vi "DP Analysis Panel.vi"(9 "Autosave? (F)":bool, 11 "Data folder in":path) -> ()   [LabVIEW 2020]
uses:
  epl-vi-lib/Utility VIs/Controls/KLegend/KLegend.xctl
  Typedefs/DP-Comparison List.ctl
  <vilib>/regexp/Match Regular Expression.xnode
panel:
  out "IOLeg":dbl(xcontrol)
  in  "Tab Control":enum32{"Isoresponse", "DP vs F2"}(tab)
  out "DPGram":cluster{"I-O Plot":dbl[], "I-O Plot":dbl[]}[](graph)
  out "DPvsFreq":cluster{"I-O Plot":dbl[], "I-O Plot":dbl[]}[](graph)
  out "DPvsF2Leg":dbl(xcontrol)
  out "exit signal":bool
  in  "Save programatically":bool
  in  "Analysis mode":enum32{"Browse", "Compare"}(tab)=enum."Compare"
  in  "Compare>":bool
  in  "File list":i32[](listbox)
  in  "Save":bool
  in  "Data folder":path
  in  "Compare list":i32[](listbox)=[0]
  in  "Criterion (dB SPL)":u16(ring)=1 items=["-5", "0", "5", "10", "15", "20", "25"]
  in  "F2 (kHz)":u16(ring) items=["5645.70", "7995.60", "11322.00", "15991.00", "22644.00", "32012.00", "45257.00", "3997.80", "5615.20", "11291.00", "22613.00"]
  in  "Exit":bool
  out "Noise Floor":i32(listbox)=2
  in  "Which DP":enum16{"2f1-f2", "f2-f1"}(ring)
  out "I-O Plot":cluster{"I-O Plot":dbl[], "I-O Plot":dbl[]}[](graph)
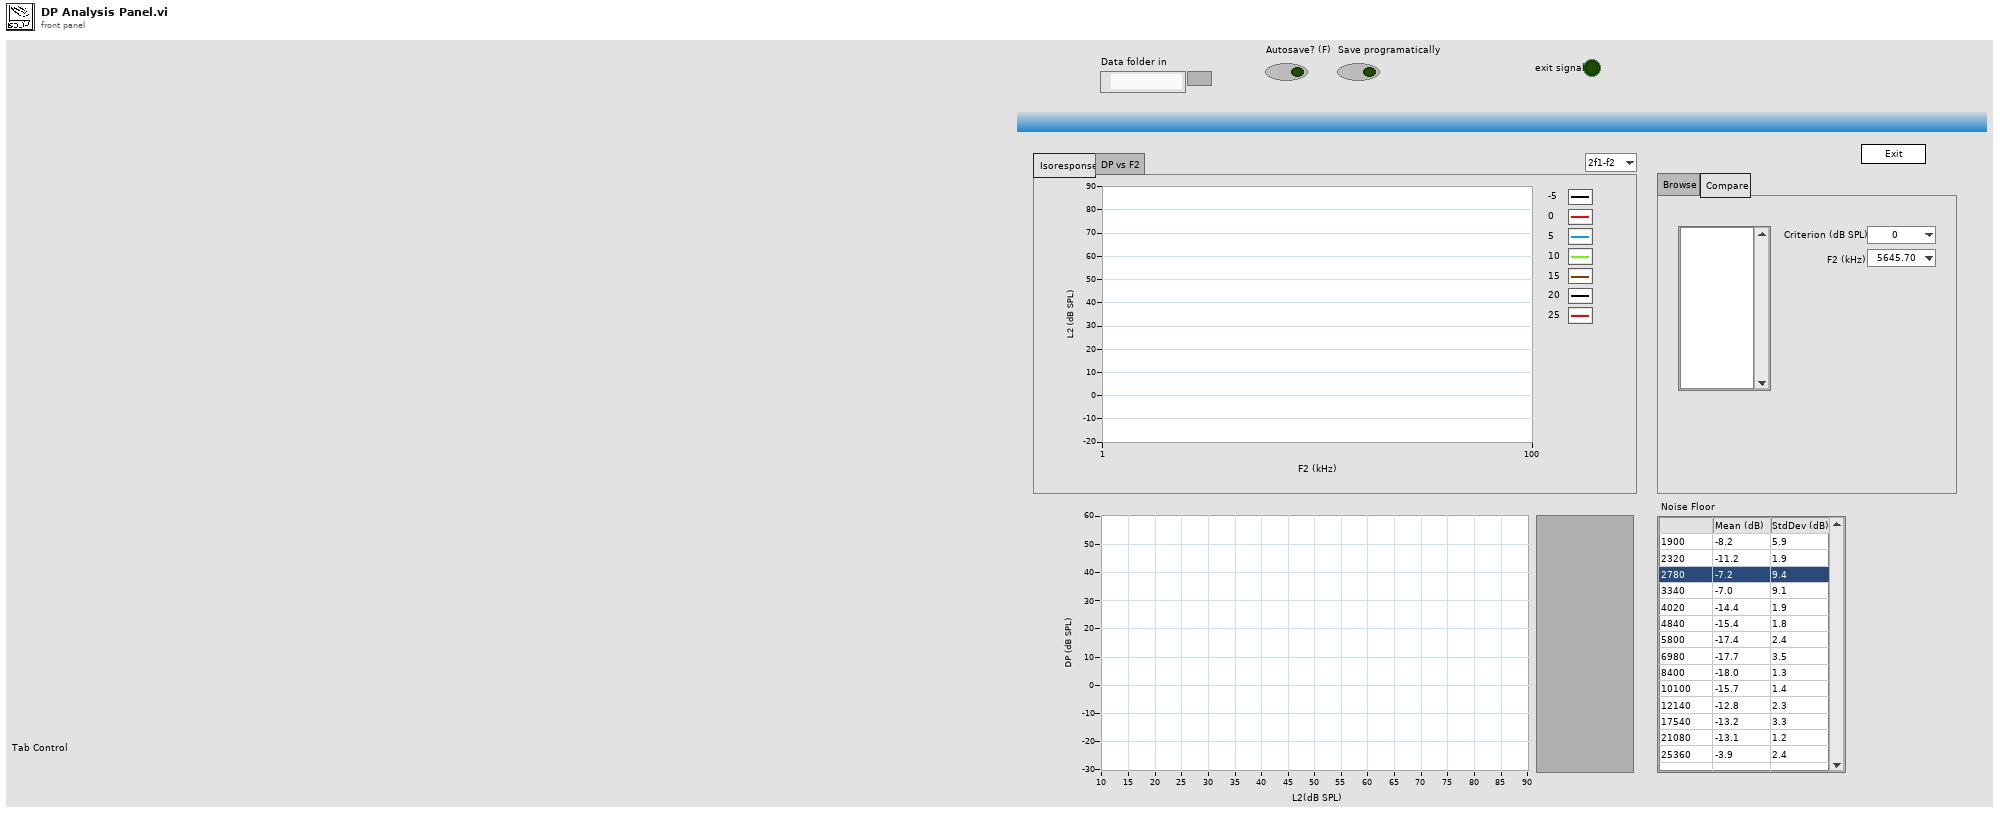
[diagram p1: front panel]
types:
  T1 = typedef "DP-Comparison List.ctl" = cluster{"Name":string, "Path":path, "Show":bool}[]
  T2 = cluster{"Array Subset":dbl[], "Array Subset":dbl[]}[]
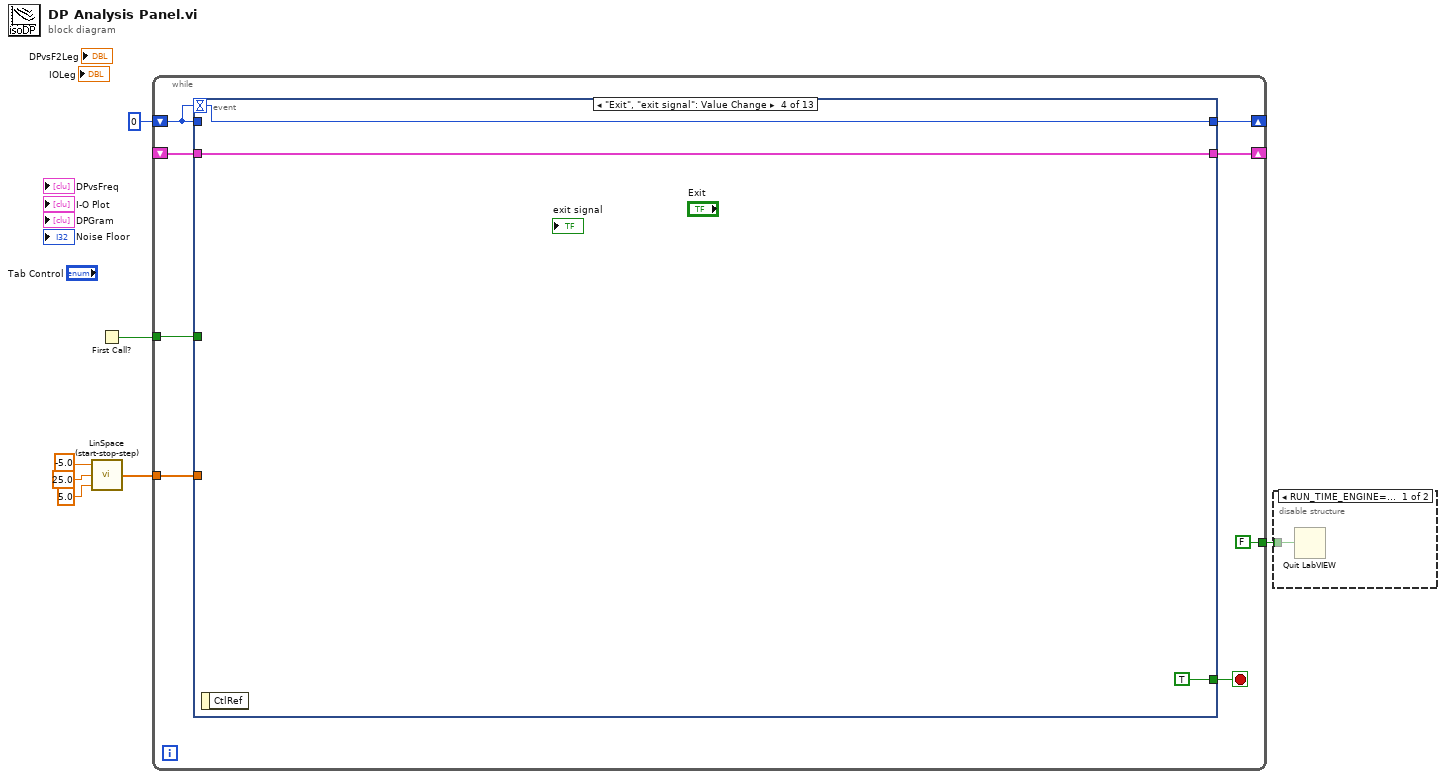
[diagram p0: block diagram]
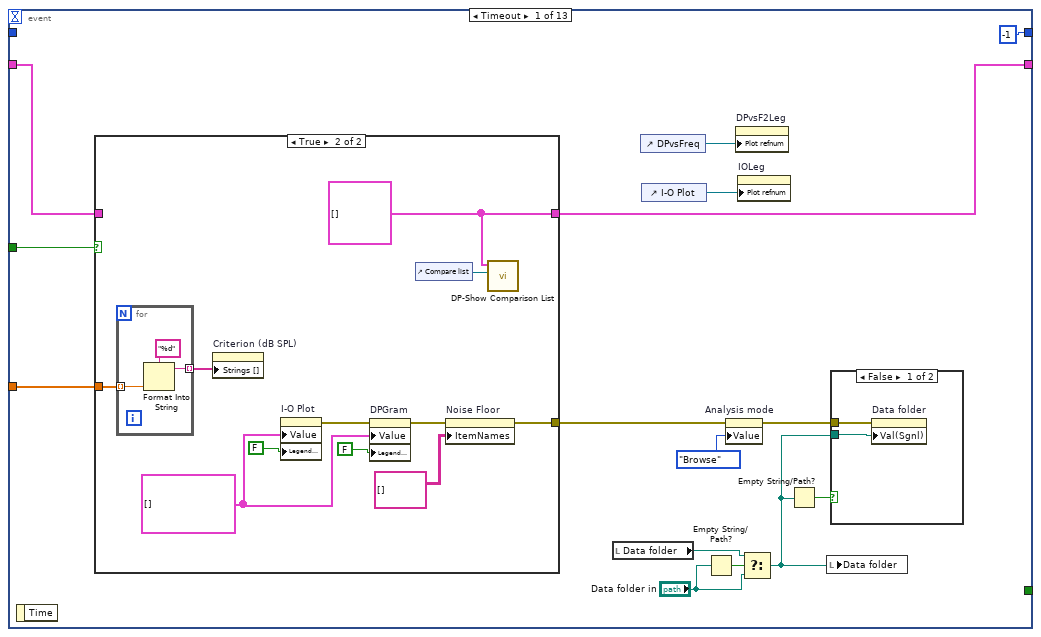
[diagram p3: hidden frame]
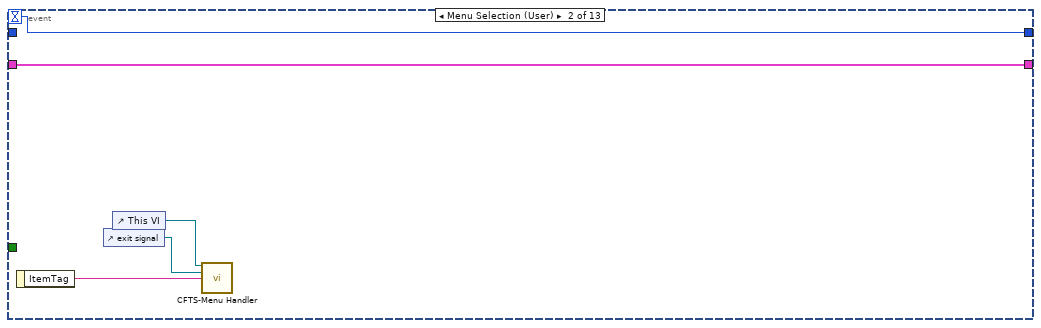
[diagram p6: hidden frame]
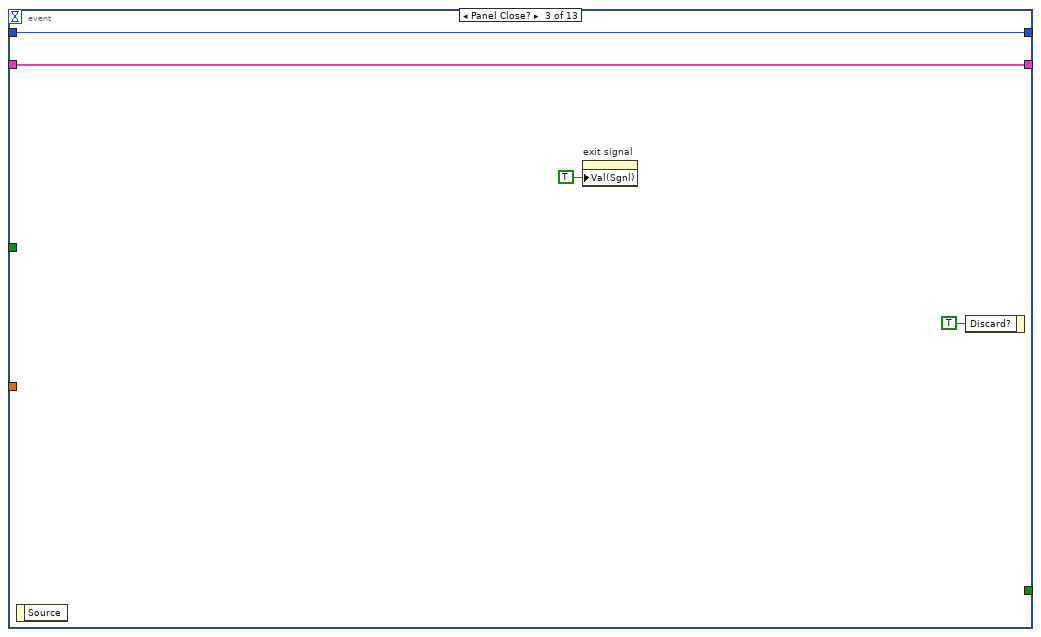
[diagram p7: hidden frame]
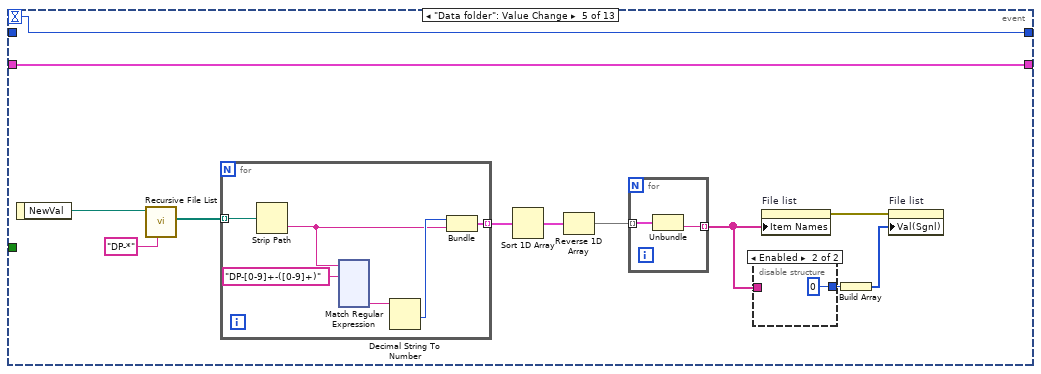
[diagram p8: hidden frame]
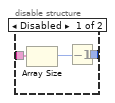
[diagram p9: hidden frame]
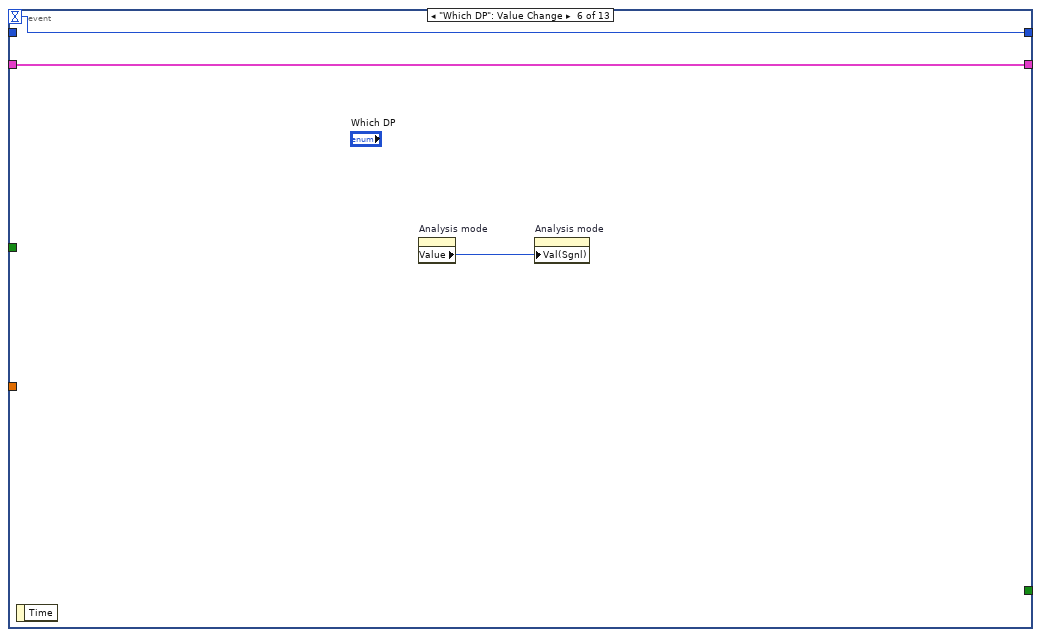
[diagram p10: hidden frame]
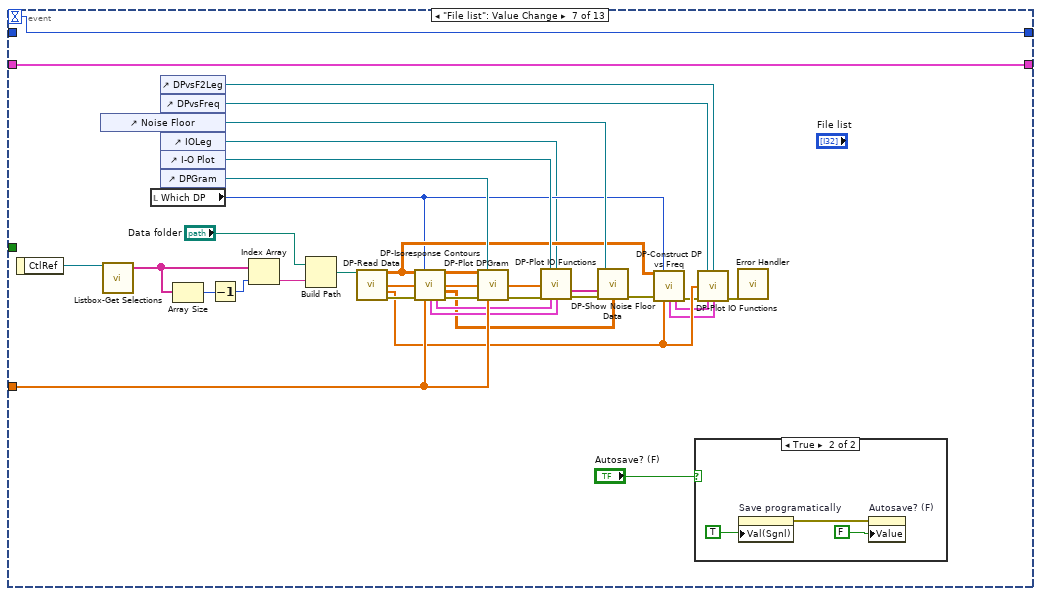
[diagram p11: hidden frame]
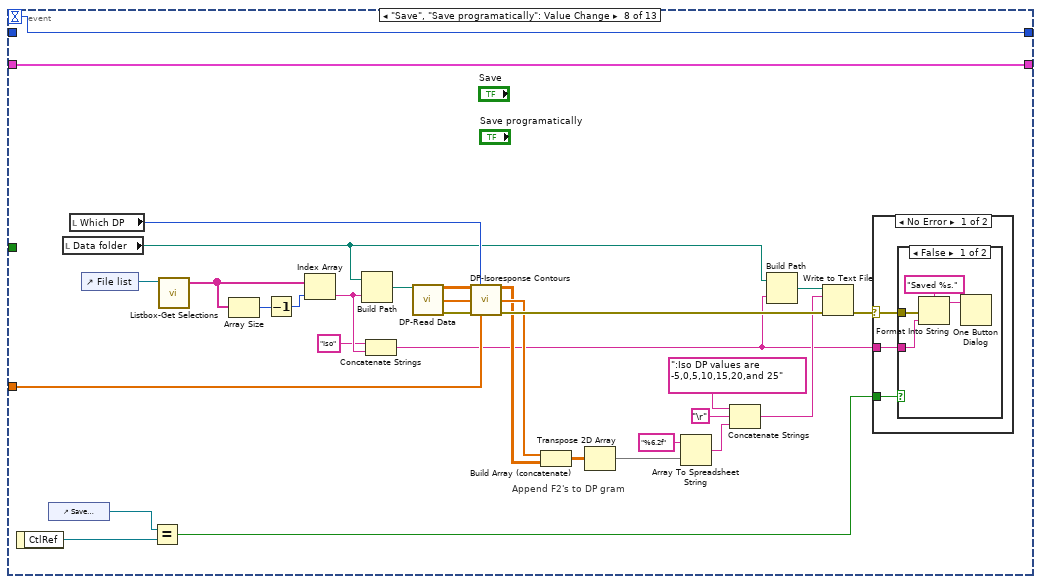
[diagram p13: hidden frame]
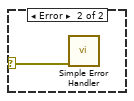
[diagram p15: hidden frame]
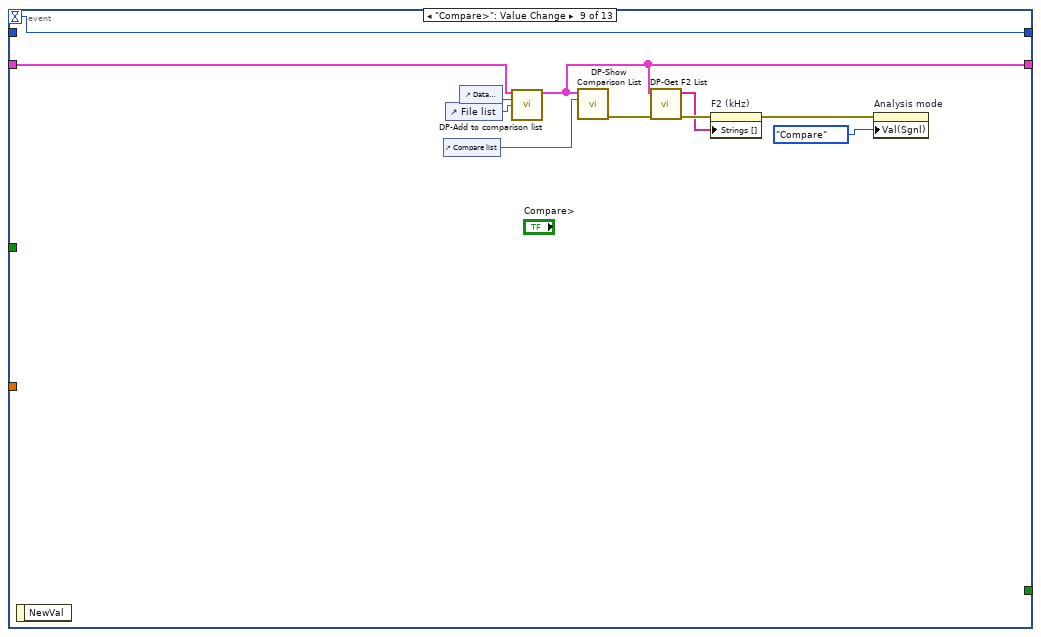
[diagram p16: hidden frame]
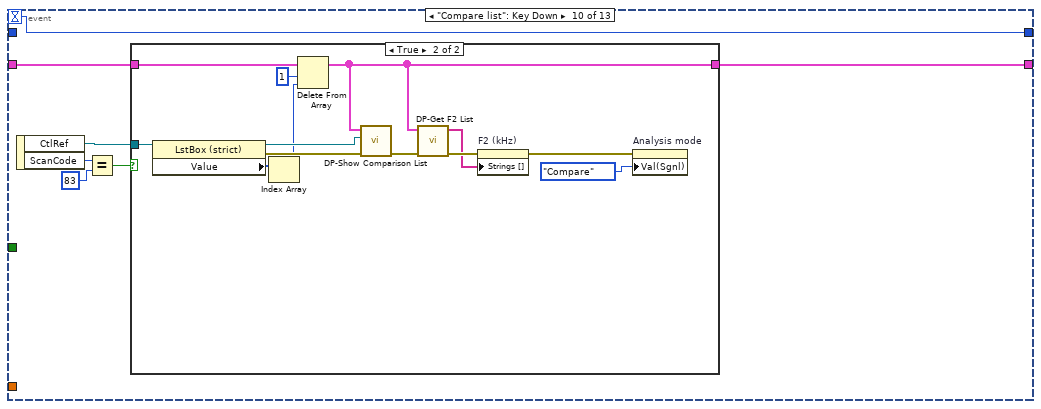
[diagram p17: hidden frame]
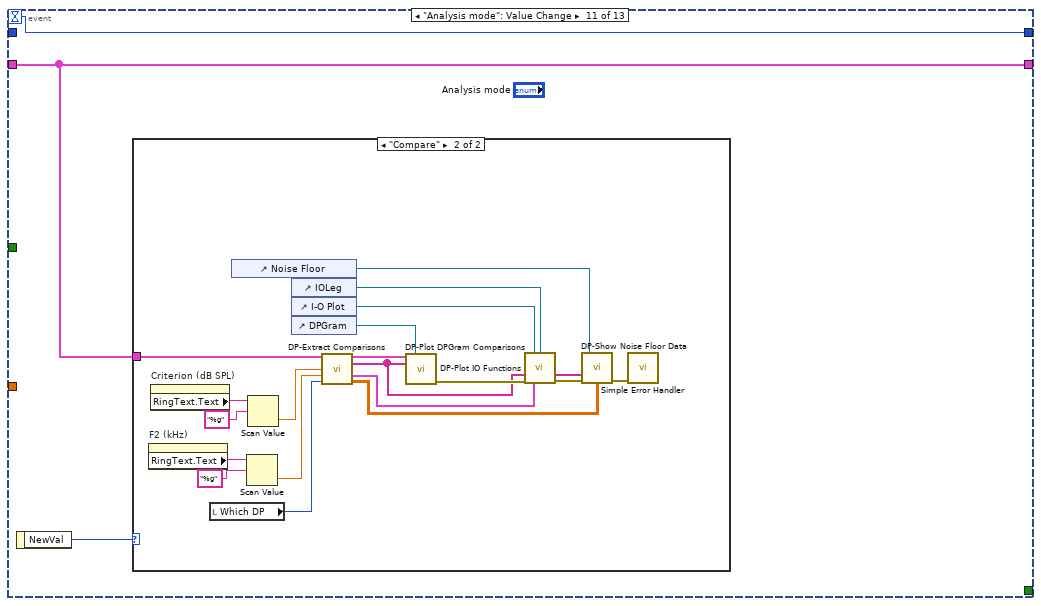
[diagram p19: hidden frame]
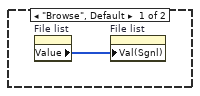
[diagram p20: hidden frame]
diagram:
  n1 = call "LinSpace (start-stop-step).vi"("Step"=5.0, "Stop"=25.0, "Start"=-5.0) -> ("Array"=w2:dbl[])  [unwired: 1 in, 1 out]
  n2 = First Call?() -> (First Call?: T/F=w6:bool)
  n3 = while {
    shift-right: [w14] -> _
    shift-left: 0 -> [w9]
    tunnel: w6 -> [w13]
    tunnel: w2 -> [w12]
    shift-right: [w11] -> _
    shift-left: _ -> [w10]
    tunnel: [FALSE] -> w1
    stop <- w15 stop-if-true
    n4 = event shown="[3] \"Exit\", \"exit signal\": Value Change" {
      selector: _ -> [_ _ _ _ _ _ _ _ _ _ _ _ _]
      dyn-events: _ -> [_ _ _ _ _ _ _ _ _ _ _ _ _]
      timeout: w9 -> [_ w49 _ w58 w71 w202 w239 w273 w291 w299 w316 w340 w351]
      tunnel: [_ _ _ TRUE _ _ _ _ _ _ _ _ _] -> w15
      tunnel: [-1 w49 w54 w58 w71 w202 w239 w273 w291 w299 w316 w340 w351] -> w14
      tunnel: w13 -> [w29 _ _ _ _ _ _ _ _ _ _ _ _]
      tunnel: w12 -> [w28 _ _ _ _ _ w234 w248 _ _ _ _ _]
      tunnel: [w27 w48 w55 w57 w67 w201 w220 w272 w284 w294 w314 w339 w343] -> w11
      tunnel: w10 -> [w26 w48 w55 w57 w67 w201 w220 w272 w282 w295 w314 w339 w347]
      tunnel: w9 -> [_ _ w54 _ _ _ _ _ _ _ _ _ _]
      event Timeout {
        n5 = event-data() -> ()  [unwired: 1 in, 1 out]
        n6 = case shown="True" w29 {
          tunnel: w28 -> [_ w38]
          tunnel: [w33 w35] -> w27
          tunnel: w26 -> [w33 _]
          tunnel: [_ w34] -> w18
          frame False {
          }
          frame True {
            w35 = T1 [] ("Comparison list")
            w42 = cluster{"I-O Plot":dbl[], "I-O Plot":dbl[]}[] [] ("I-O Plot")
            n7 = for {
              tunnel: w38 -> [w46] mode=indexing
              tunnel: [w47] -> w37 mode=indexing
              n8 = Format Into String(format string="%d", w46) -> (resulting string=w47:string)  [unwired: 2 in, 1 out]
            }
            n9 = property on="Criterion (dB SPL)" class="Ring (strict)"("Strings []"=w37) -> ()  [unwired: 2 in, 2 out]
            n10 = property on="I-O Plot" class="XYGraph (strict)"("Value"=w42, "Legend Visible"=FALSE ("Legend:Visible")) -> (error out=w43:errorcluster)  [unwired: 2 in, 1 out]
            n11 = property on="DPGram" class="XYGraph (strict)"(error in=w43, "Value"=w42, "Legend Visible"=FALSE ("Legend:Visible")) -> (error out=w40:errorcluster)  [unwired: 1 in, 1 out]
            n12 = control-ref of="Compare list"() -> (w36:refnum<vi>)
            n13 = property on="Noise Floor" class="MCListbox (strict)"(error in=w40, "ItemNames"=string[][] [] ("Item Names")) -> (error out=w34:errorcluster)  [unwired: 1 in, 1 out]
            n14 = call "DP-Show Comparison List.vi"("Listbox Ref"=w36, "Comparison list"=w35) -> ()  [unwired: 9 in, 1 out]
          }
        }
        n15 = local read "Data folder"() -> (w24:path)
        n16 = control-ref of="DPvsFreq"() -> (w17:refnum<vi>)
        n17 = control-ref of="I-O Plot"() -> (w16:refnum<vi>)
        n18 = Empty String/Path?(string/path="Data folder in") -> (empty?=w22:bool)
        n19 = property on="Analysis mode" class="TabCtl (strict)"(error in=w18, "Value"=enum32{"Browse", "Compare"}."Browse" ("Analysis mode")) -> (error out=w19:errorcluster)  [unwired: 1 in, 1 out]
        n20 = property on="DPvsF2Leg" class="KLegend (strict)"("Plot refnum"=w17) -> ()  [unwired: 2 in, 2 out]
        n21 = property on="IOLeg" class="KLegend (strict)"("Plot refnum"=w16) -> ()  [unwired: 2 in, 2 out]
        n22 = Select(t=w24, s=w22, f="Data folder in") -> (s? t:f=w25:path)
        n23 = Empty String/Path?(string/path=w25) -> (empty?=w21:bool)
        n24 = local write "Data folder"(w25) -> ()
        n25 = case shown="False" w21 {
          tunnel: w25 -> [w32 _]
          tunnel: w19 -> [w31 _]
          frame False {
            n26 = property on="Data folder" class="Path"(error in=w31, "Val(Sgnl)"=w32) -> ()  [unwired: 1 in, 2 out]
          }
          frame True {
          }
        }
      }
      event Menu Selection (User) {
        n27 = event-data() -> ("ItemTag"=w52:string)  [unwired: 1 in]
        n28 = control-ref of="exit signal"() -> (w51:refnum<vi>)
        n29 = control-ref of="This VI"() -> (w50:refnum<vi>)
        n30 = call "CFTS-Menu Handler.vi"("VI Refnum"=w50, "Return Refnum"=w51, "ItemTag"=w52) -> ()  [unwired: 11 in, 2 out]
      }
      event Panel Close? {
        n31 = event-data() -> ()  [unwired: 1 in, 1 out]
        n32 = property on="exit signal" class="Bool (strict)"("Val(Sgnl)"=TRUE ("Value (Signaling)")) -> ()  [unwired: 2 in, 2 out]
        n33 = event-data("Discard?"=TRUE) -> ()  [unwired: 1 in, 1 out]
      }
      event "Exit", "exit signal": Value Change {
        n34 = event-data() -> ()  [unwired: 1 in, 1 out]
      }
      event "Data folder": Value Change {
        n35 = event-data() -> ("NewVal"=w70:path)  [unwired: 1 in]
        n36 = call <vilib>:"Recursive File List.vi"("pattern"="DP-*", "Folder Path"=w70) -> ("All Files in Dir"=w68:path[])  [unwired: 5 in, 4 out]
        n37 = for {
          tunnel: w68 -> [w83] mode=indexing
          tunnel: [w80] -> w63 mode=indexing
          n38 = Strip Path(path=w83) -> (name=w78:string)  [unwired: 1 out]
          n39 = xnode "Match Regular Expression"("input string"=w78, "regular expression"="DP-[0-9]+-([0-9]+)") -> ("submatch 1"=w81:string)  [unwired: 4 in, 5 out]
          n40 = Decimal String To Number(string=w81) -> (number=w79:i32)  [unwired: 2 in, 1 out]
          n41 = Bundle(w79, "name"=w78) -> (w80:cluster{i32, "name":string})  [unwired: 1 in]
        }
        n42 = Sort 1D Array(array=w63) -> (sorted array=w62:cluster{i32, "name":string}[])
        n43 = Reverse 1D Array(array=w62) -> (reversed array=w60:cluster{i32, "name":string}[])
        n44 = for {
          tunnel: w60 -> [w77] mode=indexing
          tunnel: [w76] -> w61 mode=indexing
          n45 = Unbundle(w77) -> ("name"=w76:string)  [unwired: 1 out]
        }
        n46 = disable-structure shown="Enabled" {
          disable-tunnel: [w73 0] -> w65
          disable-tunnel: w61 -> [w72 _]
          frame Disabled {
            n47 = Array Size(array=w72) -> (size(s)=w74:i32)
            n48 = Decrement(x=w74) -> (x-1=w73:i32)
          }
          frame Enabled {
          }
        }
        n49 = property on="File list" class="LstBox (strict)"("Item Names"=w61) -> (error out=w66:errorcluster)  [unwired: 2 in, 1 out]
        n50 = Build Array(w65) -> (w64:i32[])
        n51 = property on="File list" class="LstBox (strict)"(error in=w66, "Val(Sgnl)"=w64) -> ()  [unwired: 1 in, 2 out]
      }
      event "Which DP": Value Change {
        n52 = event-data() -> ()  [unwired: 1 in, 1 out]
        n53 = property on="Analysis mode" class="TabCtl (strict)"() -> ("Value"=w200:enum32{"Browse", "Compare"})  [unwired: 2 in, 2 out]
        n54 = property on="Analysis mode" class="TabCtl (strict)"("Val(Sgnl)"=w200) -> ()  [unwired: 2 in, 2 out]
      }
      event "File list": Value Change {
        n55 = event-data() -> ("CtlRef"=w219:refnum<vi>)  [unwired: 1 in]
        n56 = control-ref of="Noise Floor"() -> (w236:refnum<vi>)
        n57 = call "Listbox-Get Selections.vi"("Listbox Ref"=w219) -> ("Selections"=w233:string[])  [unwired: 9 in, 1 out]
        n58 = local read "Which DP"() -> (w214:enum16{"2f1-f2", "f2-f1"})
        n59 = control-ref of="DPvsF2Leg"() -> (w211:refnum<vi>)
        n60 = control-ref of="DPvsFreq"() -> (w213:refnum<vi>)
        n61 = control-ref of="IOLeg"() -> (w210:refnum<vi>)
        n62 = control-ref of="I-O Plot"() -> (w237:refnum<vi>)
        n63 = control-ref of="DPGram"() -> (w238:refnum<vi>)
        n64 = Array Size(array=w233) -> (size(s)=w222:i32)
        n65 = Decrement(x=w222) -> (x-1=w221:i32)
        n66 = Index Array(array=w233, index=w221) -> (element=w224:string)
        n67 = Build Path(base path="Data folder", name or relative path=w224) -> (appended path=w223:path)
        n68 = call "DP-Read Data.vi"("Path"=w223) -> ("Data matrix"=w215:dbl[][], "F2 array"=w216:dbl[], "L2 array"=w212:dbl[], "error out"=w232:errorcluster)  [unwired: 11 in]
        n69 = call "DP-Isoresponse Contours.vi"("Data matrix"=w215, "Which DP"=w214, "F2 array"=w216, "error in"=w232, "criteria (dB)"=w234) -> ("DPGram"=w230:dbl[][], "F2 out"=w229:dbl[], "Noise floor data"=w203:dbl[][], "Array"=w204:T2, "IO Functions"=w226:T2, "error out"=w231:errorcluster)  [unwired: 5 in]
        n70 = call "DP-Plot DPGram.vi"("DPGram"=w230, "Plot refnum"=w238, "F2"=w229, "error in"=w231, "criteria (dB)"=w234) -> ("F2 out"=w228:dbl[], "error out"=w227:errorcluster)  [unwired: 8 in, 1 out]
        n71 = call "DP-Plot IO Functions.vi"("Plot refnum"=w237, "Legend"=w210, "Vals"=w228, "error in"=w227, "Value"=w226, "noise"=w204) -> ("Names out"=w209:string[], "error out"=w225:errorcluster)  [unwired: 8 in]
        n72 = call "DP-Show Noise Floor Data.vi"("Listbox Refnum"=w236, "Names"=w209, "error in"=w225, "Noise floor data"=w203) -> ("error out"=w217:errorcluster)  [unwired: 11 in]
        n73 = call "DP-Construct DP vs Freq.vi"("Data matrix"=w215, "Which DP"=w214, "error in"=w217, "L2 array"=w212) -> ("noise floor"=w205:T2, "IO Functions"=w208:T2, "error out"=w207:errorcluster)  [unwired: 9 in]
        n74 = case shown="True" "Autosave? (F)" {
          frame False {
          }
          frame True {
            n75 = property on="Save programatically" class="Bool (strict)"("Val(Sgnl)"=TRUE ("Value (Signaling)")) -> (error out=w241:errorcluster)  [unwired: 2 in, 1 out]
            n76 = property on="Autosave? (F)" class="Bool (strict)"(error in=w241, "Value"=FALSE ("Autosave? (F)")) -> ()  [unwired: 1 in, 2 out]
          }
        }
        n77 = call "DP-Plot IO Functions.vi"("Plot refnum"=w213, "Legend"=w211, "Vals"=w212, "error in"=w207, "Value"=w208, "noise"=w205) -> ("error out"=w206:errorcluster)  [unwired: 8 in, 1 out]
        n78 = call "Error Handler.vi"("error in (no error)"=w206) -> ()  [unwired: 13 in, 2 out]
      }
      event "Save", "Save programatically": Value Change {
        # "Append F2's to DP gram"
        n79 = event-data() -> ("CtlRef"=w244:refnum<vi>)  [unwired: 1 in]
        n80 = control-ref of="Save programatically"() -> (w245:refnum<vi>)
        n81 = local read "Data folder"() -> (w260:path)
        n82 = local read "Which DP"() -> (w264:enum16{"2f1-f2", "f2-f1"})
        n83 = control-ref of="File list"() -> (w263:refnum<vi>)
        n84 = Equal?(x=w245, y=w244) -> (x = y?=w243:bool)
        n85 = call "Listbox-Get Selections.vi"("Listbox Ref"=w263) -> ("Selections"=w271:string[])  [unwired: 9 in, 1 out]
        n86 = Array Size(array=w271) -> (size(s)=w266:i32)
        n87 = Decrement(x=w266) -> (x-1=w265:i32)
        n88 = Index Array(array=w271, index=w265) -> (element=w262:string)
        n89 = Build Path(base path=w260, name or relative path=w262) -> (appended path=w267:path)
        n90 = Concatenate Strings("Iso" ("string"), w262) -> (w246:string)
        n91 = call "DP-Read Data.vi"("Path"=w267) -> ("Data matrix"=w270:dbl[][], "F2 array"=w268:dbl[], "error out"=w269:errorcluster)  [unwired: 11 in, 1 out]
        n92 = call "DP-Isoresponse Contours.vi"("Data matrix"=w270, "Which DP"=w264, "F2 array"=w268, "error in"=w269, "criteria (dB)"=w248) -> ("DPGram"=w251:dbl[][], "F2 out"=w252:dbl[], "error out"=w254:errorcluster)  [unwired: 5 in, 3 out]
        n93 = Build Array (concatenate)(w252, w251) -> (w250:dbl[][])
        n94 = Transpose 2D Array(2D array=w250) -> (transposed array=w249:dbl[][])
        n95 = Array To Spreadsheet String(array=w249, 3:"%6.2f") -> (spreadsheet string=w259:string)  [unwired: 1 in]
        n96 = Concatenate Strings(":Iso DP values are -5,0,5,10,15,20,and 25", "\r", w259) -> (w253:string)
        n97 = Build Path(base path=w260, name or relative path=w246) -> (appended path=w255:path)
        n98 = Write to Text File(file (use dialog)=w255, text=w253, error in=w254) -> (error out=w247:errorcluster)  [unwired: 1 in, 2 out]
        n99 = case shown="No Error" w247 {
          selector: w247 -> [w276 w281]
          tunnel: w246 -> [w275 _]
          tunnel: w243 -> [w274 _]
          frame No Error {
            n100 = case shown="False" w274 {
              tunnel: w276 -> [w280 _]
              tunnel: w275 -> [w277 _]
              frame False {
                n101 = Format Into String(format string="Saved %s.", error in=w280, w277) -> (resulting string=w279:string)  [unwired: 1 in, 1 out]
                n102 = One Button Dialog(message=w279) -> ()  [unwired: 1 in, 1 out]
              }
              frame True {
              }
            }
          }
          frame Error {
            n103 = call <vilib>:"Simple Error Handler.vi"("error in (no error)"=w281) -> ()  [unwired: 4 in, 5 out]
          }
        }
      }
      event "Compare>": Value Change {
        n104 = event-data() -> ()  [unwired: 1 in, 1 out]
        n105 = control-ref of="Compare list"() -> (w285:refnum<vi>)
        n106 = control-ref of="File list"() -> (w290:refnum<vi>)
        n107 = control-ref of="Data folder"() -> (w286:refnum<vi>)
        n108 = call "DP-Add to comparison list.vi"("Comparison list"=w282, "Data folder ref"=w286, "File listbox ref"=w290) -> ("Comparison list out"=w284:T1)  [unwired: 12 in]
        n109 = call "DP-Show Comparison List.vi"("Listbox Ref"=w285, "Comparison list"=w284) -> ("error out"=w289:errorcluster)  [unwired: 9 in]
        n110 = call "DP-Get F2 List.vi"("error in (no error)"=w289, "Comparison list"=w284) -> ("error out"=w292:errorcluster, "F2 List"=w287:string[])  [unwired: 8 in]
        n111 = property on="F2 (kHz)" class="Ring (strict)"(error in=w292, "Strings []"=w287) -> (error out=w283:errorcluster)  [unwired: 1 in, 1 out]
        n112 = property on="Analysis mode" class="TabCtl (strict)"(error in=w283, "Val(Sgnl)"=enum32{"Browse", "Compare"}."Compare" ("Value (Signaling)")) -> ()  [unwired: 1 in, 2 out]
      }
      event "Compare list": Key Down {
        n113 = event-data() -> ("CtlRef"=w293:refnum<vi>, "ScanCode"=w298:i16)  [unwired: 1 in]
        n114 = Equal?(x=w298, y=i16 83) -> (x = y?=w296:bool)
        n115 = case shown="True" w296 {
          tunnel: w295 -> [w300 w313]
          tunnel: [w300 w306] -> w294
          tunnel: w293 -> [_ w305]
          frame False {
          }
          frame True {
            n116 = property class="LstBox (strict)"(reference=w305) -> (reference out=w302:refnum<vi>, error out=w303:errorcluster, "Value"=w304:i32[])  [unwired: 1 in]
            n117 = Index Array(array=w304) -> (element=w301:i32)  [unwired: 1 in]
            n118 = Delete From Array(array=w313, length=1, index=w301) -> (array with subset deleted=w306:T1)  [unwired: 1 out]
            n119 = call "DP-Show Comparison List.vi"("error in (no error)"=w303, "Listbox Ref"=w302, "Comparison list"=w306) -> ("error out"=w310:errorcluster)  [unwired: 8 in]
            n120 = call "DP-Get F2 List.vi"("error in (no error)"=w310, "Comparison list"=w306) -> ("error out"=w311:errorcluster, "F2 List"=w308:string[])  [unwired: 8 in]
            n121 = property on="F2 (kHz)" class="Ring (strict)"(error in=w311, "Strings []"=w308) -> (error out=w307:errorcluster)  [unwired: 1 in, 1 out]
            n122 = property on="Analysis mode" class="TabCtl (strict)"(error in=w307, "Val(Sgnl)"=enum32{"Browse", "Compare"}."Compare" ("Value (Signaling)")) -> ()  [unwired: 1 in, 2 out]
          }
        }
      }
      event "Analysis mode": Value Change {
        n123 = event-data() -> ("NewVal"=w315:enum32{"Browse", "Compare"})  [unwired: 1 in]
        n124 = case shown="\"Compare\"" w315 {
          tunnel: w314 -> [_ w333]
          frame "Browse", Default {
            n125 = property on="File list" class="LstBox (strict)"() -> ("Value"=w317:i32[])  [unwired: 2 in, 2 out]
            n126 = property on="File list" class="LstBox (strict)"("Val(Sgnl)"=w317) -> ()  [unwired: 2 in, 2 out]
          }
          frame "Compare" {
            n127 = property on="F2 (kHz)" class="Ring (strict)"() -> ("RingText.Text"=w326:string)  [unwired: 2 in, 2 out]
            n128 = property on="Criterion (dB SPL)" class="Ring (strict)"() -> ("RingText.Text"=w332:string)  [unwired: 2 in, 2 out]
            n129 = local read "Which DP"() -> (w329:enum16{"2f1-f2", "f2-f1"})
            n130 = control-ref of="Noise Floor"() -> (w335:refnum<vi>)
            n131 = Scan Value(string=w326, format string="%g") -> (value=w325:dbl)  [unwired: 1 in, 1 out]
            n132 = Scan Value(string=w332, format string="%g") -> (value=w330:dbl)  [unwired: 1 in, 1 out]
            n133 = control-ref of="IOLeg"() -> (w319:refnum<vi>)
            n134 = control-ref of="I-O Plot"() -> (w336:refnum<vi>)
            n135 = control-ref of="DPGram"() -> (w337:refnum<vi>)
            n136 = call "DP-Extract Comparisons.vi"("Comparison list"=w333, "Criterion"=w330, "F2 (kHz)"=w325, "Which DP"=w329) -> ("DP Plots"=w328:cluster{"F2 array":dbl[], "DPGram":dbl[]}[], "Names"=w318:string[], "IO Plots"=w323:T2, "Noise floor data"=w321:dbl[][])  [unwired: 8 in]
            n137 = call "DP-Plot DPGram Comparisons.vi"("Plots"=w328, "Plot refnum"=w337, "Names"=w318) -> ("error out"=w334:errorcluster)  [unwired: 12 in]
            n138 = call "DP-Plot IO Functions.vi"("Plot refnum"=w336, "Legend"=w319, "Names in"=w318, "error in"=w334, "Value"=w323) -> ("Names out"=w322:string[], "error out"=w324:errorcluster)  [unwired: 9 in]
            n139 = call "DP-Show Noise Floor Data.vi"("Listbox Refnum"=w335, "Names"=w322, "error in"=w324, "Noise floor data"=w321) -> ("error out"=w320:errorcluster)  [unwired: 11 in]
            n140 = call <vilib>:"Simple Error Handler.vi"("error in (no error)"=w320) -> ()  [unwired: 4 in, 5 out]
          }
        }
      }
      event "F2 (kHz)", "Criterion (dB SPL)": Value Change {
        n141 = event-data() -> ()  [unwired: 1 in, 1 out]
        n142 = property on="Analysis mode" class="TabCtl (strict)"("Val(Sgnl)"=enum32{"Browse", "Compare"}."Compare" ("Value (Signaling)")) -> ()  [unwired: 2 in, 2 out]
      }
      event "Compare list": Double Click {
        n143 = event-data() -> ("Row"=w346:i32, "CtlRef"=w341:refnum<vi>)  [unwired: 1 in]
        n144 = Index Array(array=w347, index=w346) -> (element=w349:cluster{"Name":string, "Path":path, "Show":bool})
        n145 = Unbundle By Name(w349) -> ("Show"=w350:bool)
        n146 = Not(x=w350) -> (.not. x?=w348:bool)
        n147 = Bundle By Name(cluster=w349, "Show"=w348) -> (w345:cluster{"Name":string, "Path":path, "Show":bool})
        n148 = Replace Array Subset(array=w347, new element=w345, index=w346) -> (w343:T1)
        n149 = call "DP-Show Comparison List.vi"("Listbox Ref"=w341, "Comparison list"=w343) -> ("error out"=w342:errorcluster)  [unwired: 9 in]
        n150 = property on="Analysis mode" class="TabCtl (strict)"(error in=w342, "Val(Sgnl)"=enum32{"Browse", "Compare"}."Compare" ("Value (Signaling)")) -> ()  [unwired: 1 in, 2 out]
      }
    }
  }
  n151 = disable-structure shown="RUN_TIME_ENGINE==True" {
    disable-tunnel: w1 -> [w352 _]
    frame condition #0 {
      n152 = Quit LabVIEW(quit? (T)=w352) -> ()
    }
    frame condition #1 (active) {
    }
  }
